vi "Set Remote Mode.vi"(8 "error in (no error)":errorcluster, 11 ".NET Refnum in":refnum<k24>) -> (0 "error out":errorcluster, 3 ".NET Refnum out":refnum<k24>)   [LabVIEW 2019, in "ESP301.lvlib"]
uses:
  ESP301.lvlib
  Newport.ESP301.CommandInterface
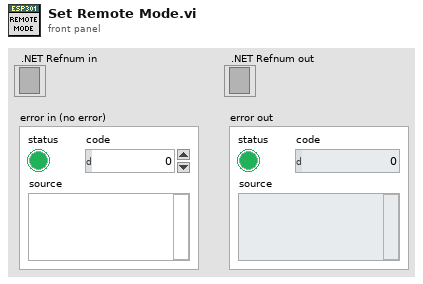
[diagram p1: front panel]
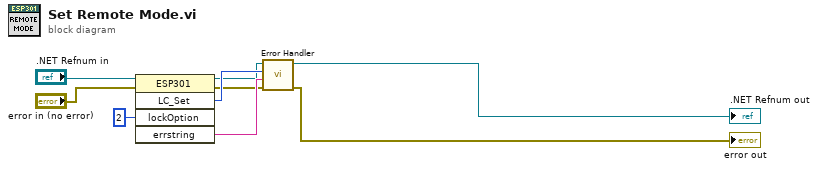
[diagram p0: block diagram]
diagram:
  n1 = invoke class="ESP301" method="LC_Set"(reference=".NET Refnum in", error in="error in (no error)", "lockOption"=2) -> (reference out=w5:refnum<k24>, error out=w2:errorcluster, "LC_Set"=w7:i32, "errstring"=w6:string)  [unwired: 2 in, 1 out]
  n2 = call "Error Handler.vi"("error in (no error)"=w2, "value"=w6, "OpenInstrument"=w7, ".NET Refnum in"=w5) -> ("error out"=→"error out":errorcluster, ".NET Refnum out"=→".NET Refnum out":refnum<k24>)  [unwired: 6 in]
